vi "options.vi"(10 "application request in":T3, 11 "http responder in":refnum<class "http responder.lvclass">) -> (2 "application response out":T1, 3 "http responder out":refnum<class "http responder.lvclass">)   [LabVIEW 2013, in "http responder.lvclass"]
uses:
  http responder.lvclass
  http request.ctl
  http method.ctl
  http response.ctl
  http response packet type.ctl
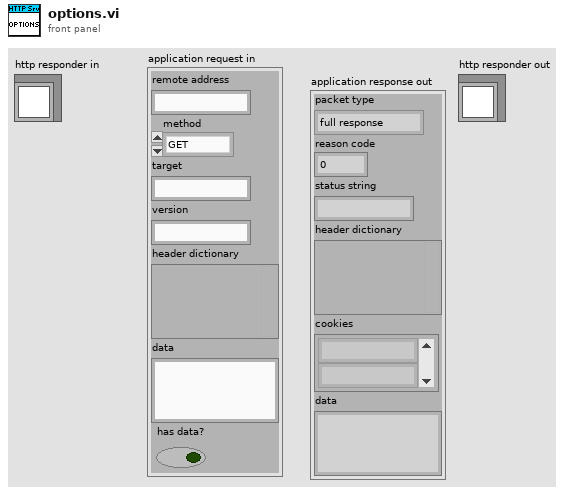
[diagram p1: front panel]
types:
  T1 = typedef "http response.ctl" = cluster{"packet type":T2, "reason code":u16, "status string":string, "header dictionary":variant, "cookies":string[], "data":string}
  T2 = typedef "http response packet type.ctl" = enum16{"full response", "header only", "data only", "last data"}
  T3 = typedef "http request.ctl" = cluster{"remote address":string, "method":T4, "target":string, "version":string, "header dictionary":variant, "data":string, "has data?":bool}
  T4 = typedef "http method.ctl" = enum16{"GET", "POST", "PUT", "DELETE", "HEAD", "OPTIONS", "upgrade"}
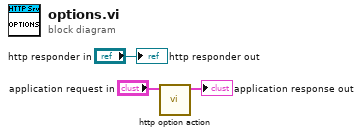
[diagram p0: block diagram]
diagram:
  n1 = call "http option action.vi"("application request in"="application request in") -> ("application request out"=→"application response out":T1)  [unwired: 10 in]
  "http responder out" <- "http responder in"
